vi "PTSequencer.set next step.vi"(0 "i ref in":refnum<vi>, 2 "passed":bool, 3 "ms timeout (10000)":i32=10000, 5 "error in (no error)":errorcluster) -> (14 "i ref out":refnum<vi>, 16 "next state":string, 17 "timed out":bool, 19 "error out":errorcluster)   [LabVIEW 2014, in "PTSequencer.lvlib"]
uses:
  PTSequencer.lvlib
  CSCore/BaseSM/BaseSM.lvlib
  CSlibraries-extern/DimLVEvent/LVDimInterface/LVDimInterface.lvlib
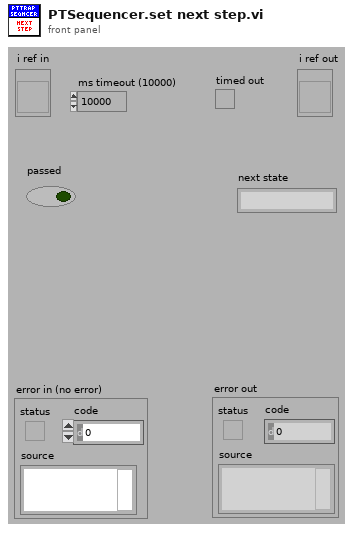
[diagram p1: front panel]
types:
  T1 = typedef "PTSequencer.lvlib/PTSequencer.i attribute.ctl" = cluster{"subsequence":bool, "mode":T2, "i step":i32, "nofLoops":i32, "i loop":i32, "Running":bool, "Paused":bool, "step done":bool, "loop done":bool, "seq done":bool, "DIM IDs":cluster{"step done":i32, "loop done":i32, "seq done":i32, "i step":i32, "i loop":i32}, "use stop conditions":bool, "stop conditions":T3[], "Step List":T5[], "DIM subsriptions":string[], "stop cond indexes":i32[], "step cond indexes":cluster{"step condition IDs":cluster{"step ID":i32, "condition ID":i32}[]}[], "Delay Start Time":timestamp, "status":string, "stopping":bool}
  T2 = typedef "PTSequencer.lvlib/PTSequencer.mode.ctl" = enum16{"single", "loop", "for loop"}
  T3 = typedef "PTSequencer.lvlib/PTSequencer.DIM service condition.ctl" = cluster{"DIM service":string, "descr":string, "nomValue":T4, "actValue":T4, "matched":bool, "DIM Status":cluster{"no link":bool, "quality":i32, "Time Stamp":timestamp}}
  T4 = typedef "CoreDefs.rawDataType.ctl" = i8[]
  T5 = typedef "PTSequencer.lvlib/PTSequencer.step.ctl" = cluster{"description":string, "object parameters":cluster{"object":string, "selector":string, "descriptor":string, "data":T4, "subsequence":bool, "call mode":enum16{"Simple DIM", "Synchronous"}, "data in":T4}, "result action":cluster{"check":bool, "passed":enum16{"Next", "Previous", "Repeat", "Jump"}, "failed":enum16{"Next", "Previous", "Repeat", "Jump"}, "jumpID_passed":i32, "jumpID_failed":i32}, "conditions":T3[], "fulfilled ":bool, "use delay":bool, "delay time (s)":dbl, "ID":i32}
  T6 = typedef "BaseSM.lvlib/BaseSM.i attribute.ctl" = cluster{"stateError":i32, "stateStatus":string, "stateQuality":T7, "ProcStateRef":refnum<vi>, "thread ref":refnum<vi>, "actState":string, "reqState":string, "SMQueue":refnum<queue>, "stateErrorID":i32, "stateStatusID":i32}
  T7 = typedef "BaseSM.lvlib/BaseSM.stateQuality.ctl" = i16
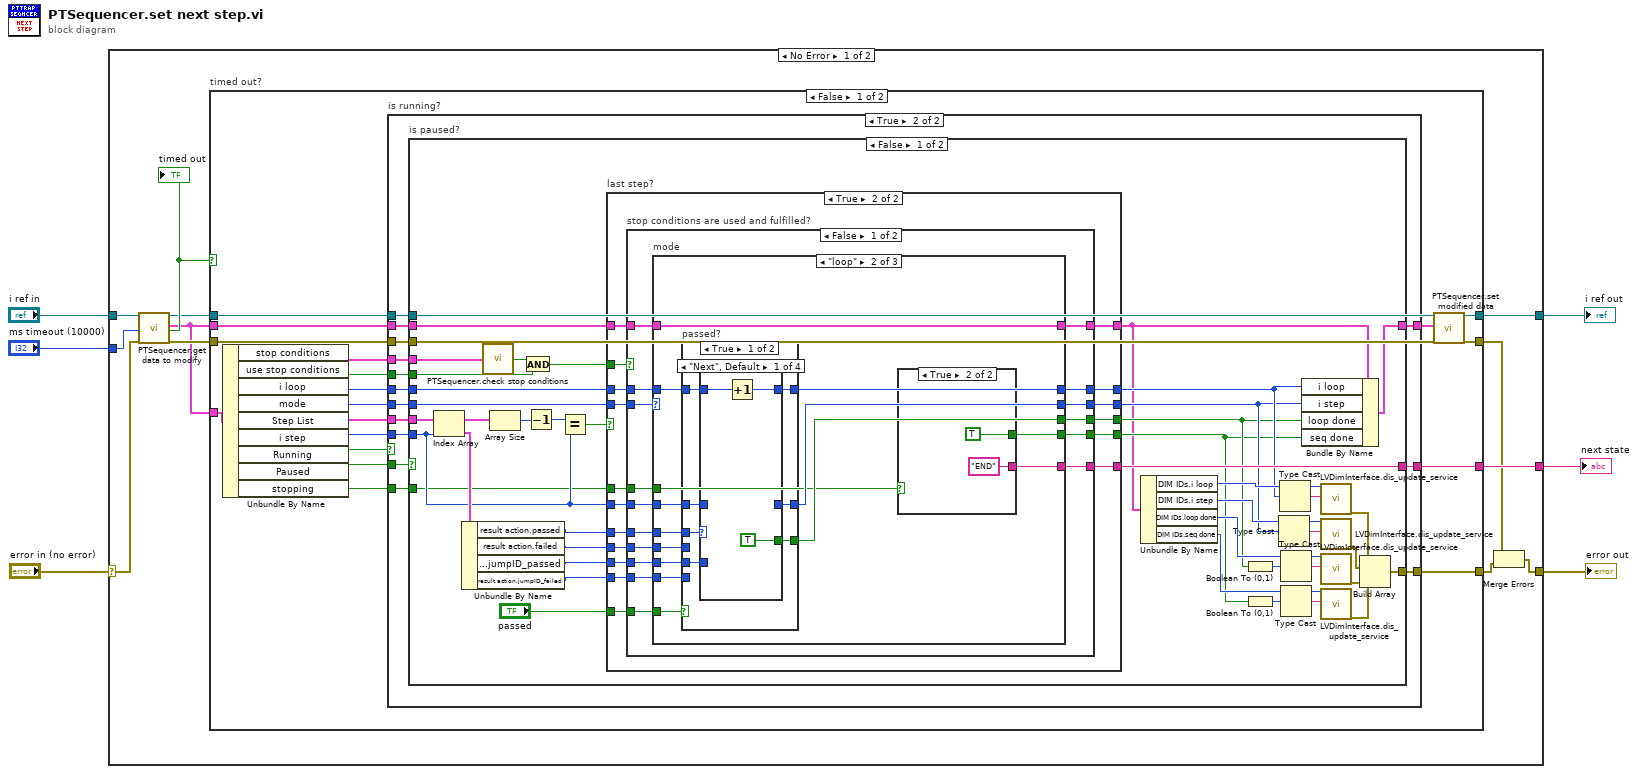
[diagram p0: block diagram]
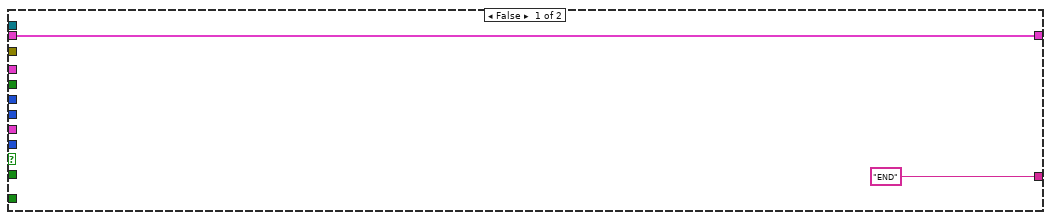
[diagram p2: hidden frame]
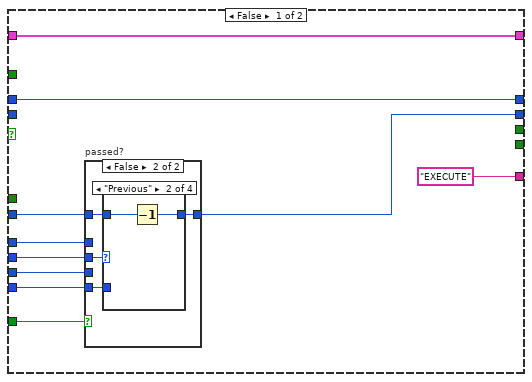
[diagram p3: hidden frame]
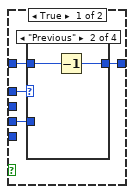
[diagram p4: hidden frame]
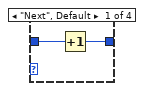
[diagram p5: hidden frame]
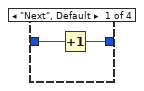
[diagram p8: hidden frame]
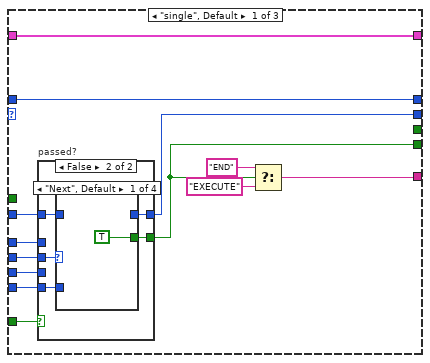
[diagram p11: hidden frame]
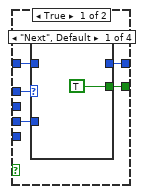
[diagram p12: hidden frame]
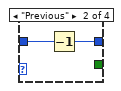
[diagram p13: hidden frame]
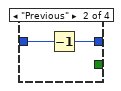
[diagram p16: hidden frame]
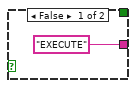
[diagram p19: hidden frame]
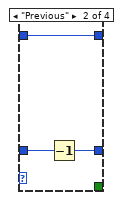
[diagram p20: hidden frame]
diagram:
  n1 = case shown="No Error" "error in (no error)" {
    selector: "error in (no error)" -> [w17 w325]
    tunnel: "i ref in" -> [w18 w324]
    tunnel: [w13 w324] -> w4
    tunnel: [w9 w325] -> w3
    tunnel: [w11 "END"] -> w2
    tunnel: "ms timeout (10000)" -> [w10 _]
    frame No Error {
      n2 = call "PTSequencer.get data to modify.vi"("i ref in"=w18, "ms timeout (10000)"=w10, "error in (no error)"=w17) -> ("i ref out"=w15:refnum<vi>, "i attribute"=w12:T1, "timed out"=w16:bool, "error out"=w14:errorcluster)  [unwired: 13 in]
      "timed out" <- w16
      n3 = case "timed out?" shown="False" w16 {
        tunnel: w12 -> [w36 _]
        tunnel: [w28 w319] -> w11
        tunnel: w15 -> [w21 w321]
        tunnel: w14 -> [w20 w320]
        tunnel: [w35 w318] -> w13
        tunnel: [w34 w317] -> w7
        tunnel: w12 -> [w24 _]
        tunnel: [w25 _] -> w8
        frame False {
          n4 = Unbundle By Name(w36) -> ("stop conditions"=w27:T3[], "use stop conditions"=w26:bool, "i loop"=w29:i32, "mode"=w30:T2, "Step List"=w32:T5[], "i step"=w31:i32, "Running"=w23:bool, "Paused"=w22:bool, "stopping"=w19:bool)
          n5 = case "is running?" shown="True" w23 {
            tunnel: [w38 w52] -> w33
            tunnel: w32 -> [_ w51]
            tunnel: w31 -> [_ w50]
            tunnel: w30 -> [_ w49]
            tunnel: w29 -> [_ w48]
            tunnel: ["END" w47] -> w28
            tunnel: w27 -> [_ w46]
            tunnel: w26 -> [_ w45]
            tunnel: [_ w44] -> w25
            tunnel: w24 -> [w38 w43]
            tunnel: w22 -> [_ w42]
            tunnel: w21 -> [_ w41]
            tunnel: w20 -> [_ w40]
            tunnel: w19 -> [_ w39]
            frame False {
            }
            frame True {
              n6 = case "is paused?" shown="False" w42 {
                tunnel: [w93 w314] -> w52
                tunnel: w51 -> [w91 _]
                tunnel: w50 -> [w56 _]
                tunnel: w49 -> [w87 _]
                tunnel: w48 -> [w86 _]
                tunnel: [w85 w312] -> w47
                tunnel: w46 -> [w84 _]
                tunnel: w45 -> [w82 _]
                tunnel: [w62 w310] -> w44
                tunnel: w43 -> [w61 w314]
                tunnel: w41 -> [_ w316]
                tunnel: w40 -> [_ w315]
                tunnel: w39 -> [w53 _]
                frame False {
                  n7 = Index Array(array=w91, index=w56) -> (element=w92:T5)
                  n8 = Unbundle By Name(w92) -> ("result action.passed"=w59:enum16{"Next", "Previous", "Repeat", "Jump"}, "result action.failed"=w58:enum16{"Next", "Previous", "Repeat", "Jump"}, "result action.jumpID_passed"=w57:i32, "result action.jumpID_failed"=w54:i32)
                  n9 = call "PTSequencer.check stop conditions.vi"("conditions"=w84) -> ("fulfilled"=w83:bool)
                  n10 = Array Size(array=w91) -> (size(s)=w90:i32)
                  n11 = And(x=w83, y=w82) -> (x .and. y?=w81:bool)
                  n12 = Decrement(x=w90) -> (x-1=w89:i32)
                  n13 = Equal?(x=w89, y=w56) -> (x = y?=w88:bool)
                  n14 = case "last step?" shown="True" w88 {
                    tunnel: w87 -> [_ w140]
                    tunnel: [w103 w137] -> w72
                    tunnel: w86 -> [w103 w134]
                    tunnel: ["EXECUTE" w133] -> w85
                    tunnel: w81 -> [_ w139]
                    tunnel: [w99 w138] -> w71
                    tunnel: [_ w136] -> w68
                    tunnel: [_ w135] -> w67
                    tunnel: w61 -> [w101 w132]
                    tunnel: [w101 w131] -> w60
                    tunnel: w59 -> [w98 w128]
                    tunnel: w58 -> [w97 w127]
                    tunnel: w57 -> [w96 w126]
                    tunnel: w56 -> [w100 w130]
                    tunnel: "passed" -> [w95 w129]
                    tunnel: w54 -> [w94 w125]
                    tunnel: w53 -> [_ w124]
                    frame False {
                      n15 = case "passed?" shown="False" w95 {
                        tunnel: w100 -> [w107 w117]
                        tunnel: w96 -> [w106 _]
                        tunnel: w97 -> [_ w115]
                        tunnel: w98 -> [w105 _]
                        tunnel: [w104 w116] -> w99
                        tunnel: w94 -> [_ w114]
                        frame True {
                          n16 = case shown="\"Previous\"" w105 {
                            tunnel: w107 -> [w109 w111 w112 _]
                            tunnel: w106 -> [_ _ _ w113]
                            tunnel: [w108 w110 w112 w113] -> w104
                            frame "Next", Default {
                              n17 = Increment(x=w109) -> (x+1=w108:i32)
                            }
                            frame "Previous" {
                              n18 = Decrement(x=w111) -> (x-1=w110:i32)
                            }
                            frame "Repeat" {
                            }
                            frame "Jump" {
                            }
                          }
                        }
                        frame False {
                          n19 = case shown="\"Previous\"" w115 {
                            tunnel: w117 -> [w119 w121 w122 _]
                            tunnel: [w118 w120 w122 w123] -> w116
                            tunnel: w114 -> [_ _ _ w123]
                            frame "Next", Default {
                              n20 = Increment(x=w119) -> (x+1=w118:i32)
                            }
                            frame "Previous" {
                              n21 = Decrement(x=w121) -> (x-1=w120:i32)
                            }
                            frame "Repeat" {
                            }
                            frame "Jump" {
                            }
                          }
                        }
                      }
                    }
                    frame True {
                      n22 = case "stop conditions are used and fulfilled?" shown="False" w139 {
                        tunnel: w140 -> [w148 _]
                        tunnel: w130 -> [w152 w305]
                        tunnel: [w146 w305] -> w138
                        tunnel: [w147 w306] -> w137
                        tunnel: [w144 w309] -> w136
                        tunnel: [w143 w309] -> w135
                        tunnel: w134 -> [w149 w306]
                        tunnel: [w145 "END"] -> w133
                        tunnel: w132 -> [w151 w307]
                        tunnel: [w150 w307] -> w131
                        tunnel: w129 -> [w156 _]
                        tunnel: w128 -> [w155 _]
                        tunnel: w127 -> [w154 _]
                        tunnel: w126 -> [w153 _]
                        tunnel: w125 -> [w142 _]
                        tunnel: w124 -> [w141 _]
                        frame False {
                          n23 = case "mode" shown="\"loop\"" w148 {
                            tunnel: w151 -> [w161 w203 w252]
                            tunnel: [w161 w203 w252] -> w150
                            tunnel: w156 -> [w169 w202 w260]
                            tunnel: w142 -> [w168 w197 w255]
                            tunnel: w153 -> [w167 w198 w256]
                            tunnel: w155 -> [w165 w200 w258]
                            tunnel: w152 -> [w164 w201 w259]
                            tunnel: w154 -> [w166 w199 w257]
                            tunnel: [w157 w196 w249] -> w145
                            tunnel: [w159 w191 w248] -> w143
                            tunnel: [w163 w194 w244] -> w146
                            tunnel: [w162 w192 w251] -> w147
                            tunnel: w149 -> [w162 w193 w254]
                            tunnel: [_ w195 w247] -> w144
                            tunnel: w141 -> [_ w190 w242]
                            frame "single", Default {
                              n24 = case "passed?" shown="False" w169 {
                                tunnel: w164 -> [w174 w184]
                                tunnel: w167 -> [w173 _]
                                tunnel: w166 -> [_ w182]
                                tunnel: w165 -> [w172 _]
                                tunnel: [w171 w183] -> w163
                                tunnel: w168 -> [_ w181]
                                tunnel: [w170 w180] -> w159
                                frame True {
                                n25 = case shown="\"Next\", Default" w172 {
                                tunnel: w174 -> [_ w177 w178 _]
                                tunnel: w173 -> [_ _ _ w179]
                                tunnel: [_ w176 w178 w179] -> w171
                                tunnel: [TRUE _ _ _] -> w170
                                frame "Next", Default {
                                }
                                frame "Previous" {
                                n26 = Decrement(x=w177) -> (x-1=w176:i32)
                                }
                                frame "Repeat" {
                                }
                                frame "Jump" {
                                }
                                }
                                }
                                frame False {
                                n27 = case shown="\"Next\", Default" w182 {
                                tunnel: w184 -> [_ w187 w188 _]
                                tunnel: [_ w186 w188 w189] -> w183
                                tunnel: w181 -> [_ _ _ w189]
                                tunnel: [TRUE _ _ _] -> w180
                                frame "Next", Default {
                                }
                                frame "Previous" {
                                n28 = Decrement(x=w187) -> (x-1=w186:i32)
                                }
                                frame "Repeat" {
                                }
                                frame "Jump" {
                                }
                                }
                                }
                              }
                              n29 = Select(t="END", s=w159, f="EXECUTE") -> (s? t:f=w157:string)
                            }
                            frame "loop" {
                              n30 = case "passed?" shown="True" w202 {
                                tunnel: w201 -> [w213 w230]
                                tunnel: w198 -> [w212 _]
                                tunnel: w199 -> [_ w228]
                                tunnel: w200 -> [w211 _]
                                tunnel: [w210 w229] -> w194
                                tunnel: w197 -> [_ w227]
                                tunnel: [w209 w226] -> w195
                                tunnel: w193 -> [w208 w225]
                                tunnel: [w207 w224] -> w192
                                frame True {
                                n31 = case shown="\"Next\", Default" w211 {
                                tunnel: w213 -> [_ w219 w221 _]
                                tunnel: w212 -> [_ _ _ w223]
                                tunnel: [_ w218 w221 w223] -> w210
                                tunnel: [TRUE _ _ _] -> w209
                                tunnel: w208 -> [w215 w217 w220 w222]
                                tunnel: [w214 w217 w220 w222] -> w207
                                frame "Next", Default {
                                n32 = Increment(x=w215) -> (x+1=w214:i32)
                                }
                                frame "Previous" {
                                n33 = Decrement(x=w219) -> (x-1=w218:i32)
                                }
                                frame "Repeat" {
                                }
                                frame "Jump" {
                                }
                                }
                                }
                                frame False {
                                n34 = case shown="\"Jump\"" w228 {
                                tunnel: w230 -> [_ w236 w238 _]
                                tunnel: [_ w235 w238 w240] -> w229
                                tunnel: w227 -> [_ _ _ w240]
                                tunnel: [TRUE _ _ _] -> w226
                                tunnel: w225 -> [w232 w234 w237 w239]
                                tunnel: [w231 w234 w237 w239] -> w224
                                frame "Next", Default {
                                n35 = Increment(x=w232) -> (x+1=w231:i32)
                                }
                                frame "Previous" {
                                n36 = Decrement(x=w236) -> (x-1=w235:i32)
                                }
                                frame "Repeat" {
                                }
                                frame "Jump" {
                                }
                                }
                                }
                              }
                              n37 = case shown="True" w190 {
                                tunnel: ["EXECUTE" "END"] -> w196
                                tunnel: [_ TRUE] -> w191
                                frame False {
                                }
                                frame True {
                                }
                              }
                            }
                            frame "for loop" {
                              n38 = case "passed?" shown="True" w260 {
                                tunnel: w259 -> [w277 w294]
                                tunnel: w256 -> [w276 _]
                                tunnel: w257 -> [_ w292]
                                tunnel: w258 -> [w275 _]
                                tunnel: [w274 w293] -> w245
                                tunnel: w255 -> [_ w291]
                                tunnel: [w273 w290] -> w246
                                tunnel: w254 -> [w272 w289]
                                tunnel: [w271 w288] -> w250
                                frame True {
                                n39 = case shown="\"Jump\"" w275 {
                                tunnel: w277 -> [_ w283 w285 _]
                                tunnel: w276 -> [_ _ _ w287]
                                tunnel: [_ w282 w285 w287] -> w274
                                tunnel: [TRUE _ _ _] -> w273
                                tunnel: w272 -> [w279 w281 w284 w286]
                                tunnel: [w278 w281 w284 w286] -> w271
                                frame "Next", Default {
                                n40 = Increment(x=w279) -> (x+1=w278:i32)
                                }
                                frame "Previous" {
                                n41 = Decrement(x=w283) -> (x-1=w282:i32)
                                }
                                frame "Repeat" {
                                }
                                frame "Jump" {
                                }
                                }
                                }
                                frame False {
                                n42 = case shown="\"Jump\"" w292 {
                                tunnel: w294 -> [_ w300 w302 _]
                                tunnel: [_ w299 w302 w304] -> w293
                                tunnel: w291 -> [_ _ _ w304]
                                tunnel: [TRUE _ _ _] -> w290
                                tunnel: w289 -> [w296 w298 w301 w303]
                                tunnel: [w295 w298 w301 w303] -> w288
                                frame "Next", Default {
                                n43 = Increment(x=w296) -> (x+1=w295:i32)
                                }
                                frame "Previous" {
                                n44 = Decrement(x=w300) -> (x-1=w299:i32)
                                }
                                frame "Repeat" {
                                }
                                frame "Jump" {
                                }
                                }
                                }
                              }
                              n45 = Unbundle By Name(w252) -> ("nofLoops"=w253:i32)
                              n46 = Less Or Equal?(x=w253, y=w250) -> (x <= y?=w243:bool)
                              n47 = Or(x=w243, y=w242) -> (x .or. y?=w241:bool)
                              n48 = case shown="True" w241 {
                                tunnel: w250 -> [w263 w269]
                                tunnel: ["EXECUTE" "END"] -> w249
                                tunnel: [w263 w268] -> w251
                                tunnel: [_ TRUE] -> w248
                                tunnel: [w262 w266] -> w247
                                tunnel: w246 -> [w262 w266]
                                tunnel: w245 -> [w261 w265]
                                tunnel: [w261 w265] -> w244
                                frame False {
                                }
                                frame True {
                                n49 = Decrement(x=w269) -> (x-1=w268:i32)
                                }
                              }
                            }
                          }
                        }
                        frame True {
                          w309 = TRUE
                        }
                      }
                    }
                  }
                  n50 = Unbundle By Name(w60) -> ("DIM IDs.i loop"=w80:i32, "DIM IDs.i step"=w79:i32, "DIM IDs.loop done"=w78:i32, "DIM IDs.seq done"=w77:i32)
                  n51 = Boolean To (0,1)(Boolean=w68) -> (0, 1=w70:i16)
                  n52 = Boolean To (0,1)(Boolean=w67) -> (0, 1=w69:i16)
                  n53 = Type Cast(x=w71) -> (*(type *) &x=w75:string)  [unwired: 1 in]
                  n54 = Type Cast(x=w72) -> (*(type *) &x=w76:string)  [unwired: 1 in]
                  n55 = Type Cast(x=w70) -> (*(type *) &x=w74:string)  [unwired: 1 in]
                  n56 = Type Cast(x=w69) -> (*(type *) &x=w73:string)  [unwired: 1 in]
                  n57 = Bundle By Name(cluster=w60, "i loop"=w72, "i step"=w71, "loop done"=w68, "seq done"=w67) -> (w93:T1)
                  n58 = call "LVDimInterface.dis_update_service.vi"("my_serviceID"=w80, "data"=w76) -> ("error out"=w66:errorcluster)  [unwired: 15 in, 2 out]
                  n59 = call "LVDimInterface.dis_update_service.vi"("my_serviceID"=w79, "data"=w75) -> ("error out"=w65:errorcluster)  [unwired: 15 in, 2 out]
                  n60 = call "LVDimInterface.dis_update_service.vi"("my_serviceID"=w78, "data"=w74) -> ("error out"=w64:errorcluster)  [unwired: 15 in, 2 out]
                  n61 = call "LVDimInterface.dis_update_service.vi"("my_serviceID"=w77, "data"=w73) -> ("error out"=w63:errorcluster)  [unwired: 15 in, 2 out]
                  n62 = Build Array(w66, w65, w64, w63) -> (w62:errorcluster[])
                }
                frame True {
                  n63 = call "BaseSM.get i attribute.vi"("i ref in"=w316, "error in (no error)"=w315) -> ("i attribute"=w313:T6, "error out"=w311:errorcluster)  [unwired: 15 in, 1 out]
                  n64 = Unbundle By Name(w313) -> ("actState"=w312:string)
                  n65 = Build Array(w311) -> (w310:errorcluster[])
                }
              }
            }
          }
          n66 = call "PTSequencer.set modified data.vi"("i ref in"=w21, "CLASS.i attribute"=w33, "error in (no error)"=w20) -> ("i ref out"=w35:refnum<vi>, "error out"=w34:errorcluster)  [unwired: 15 in]
        }
        frame True {
          n67 = call "BaseSM.get i attribute.vi"("i ref in"=w321, "error in (no error)"=w320) -> ("i ref out"=w318:refnum<vi>, "i attribute"=w322:T6, "error out"=w317:errorcluster)  [unwired: 15 in]
          n68 = Unbundle By Name(w322) -> ("actState"=w319:string)
        }
      }
      n69 = Merge Errors(w7, w8) -> (w9:errorcluster)
    }
    frame Error {
    }
  }
  "i ref out" <- w4
  "error out" <- w3
  "next state" <- w2
